vi "from_boolean.vi"(8 "error in (no error)":errorcluster, 10 "value":bool) -> (0 "error out":errorcluster, 3 "Item out":refnum<class "Item.lvclass">)   [LabVIEW 2020, in "toml_edit.lvlib" / "Item.lvclass"]
uses:
  Item.lvclass
  Item.lvclass/Item.ctl
  dragon_toml_64.dll
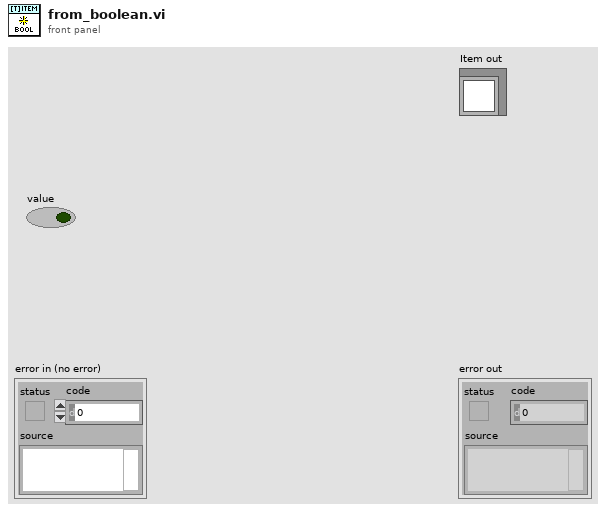
[diagram p1: front panel]
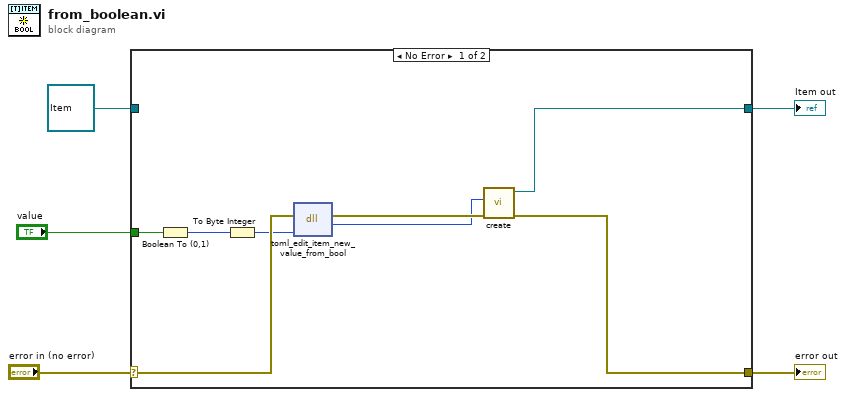
[diagram p0: block diagram]
diagram:
  n1 = case shown="No Error" "error in (no error)" {
    selector: "error in (no error)" -> [w10 w15]
    tunnel: [w9 w15] -> w4
    tunnel: [w13 w14] -> w2
    tunnel: refnum<class "Item.lvclass"> refnum ("Item in") -> [_ w14]
    tunnel: "value" -> [w12 _]
    frame No Error {
      n2 = Boolean To (0,1)(Boolean=w12) -> (0, 1=w8:i16)
      n3 = To Byte Integer(number=w8) -> (8bit integer=w6:i8)
      n4 = dll-call lib="C:/Projects/labview-project-load-tools/source/submodules/toml-edit-labview/lv_src/dragon_toml_*.*" fn="toml_edit_item_new_value_from_bool"(error in=w10, "boolean_as_i8"=w6) -> (error out=w11:errorcluster, "item_ref"=w7:u64)  [unwired: 3 in, 1 out]
      n5 = call "create.vi"("error in (no error)"=w11, "ref"=w7) -> ("error out"=w9:errorcluster, "Item out"=w13:refnum<class "Item.lvclass">)  [unwired: 7 in, 1 out]
    }
    frame Error {
    }
  }
  "error out" <- w4
  "Item out" <- w2
